vi "CorrectResponse.vi"(8 "error in (no error)":errorcluster, 11 "TrialBasedExperiment in":refnum<class "EyeCalibration.lvclass">) -> (0 "error out":errorcluster, 3 "TrialBasedExperiment out":refnum<class "EyeCalibration.lvclass">)   [LabVIEW 2014, in "EyeCalibration.lvclass"]
uses:
  EyeCalibration.lvclass
  Trial Based Experiment Statechart/MatlabExperiment/MatlabExperiment.lvclass
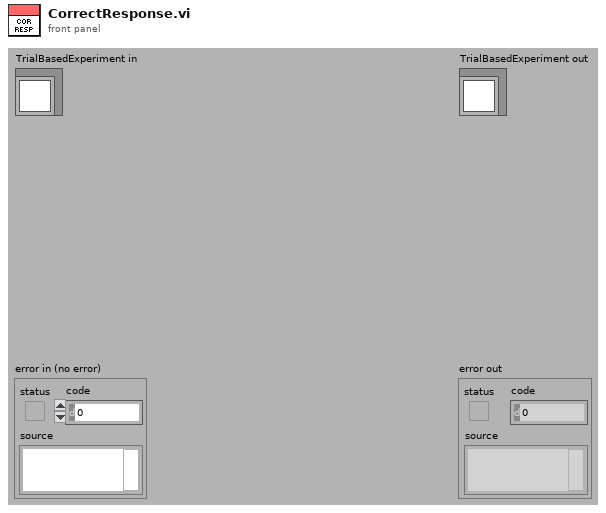
[diagram p1: front panel]
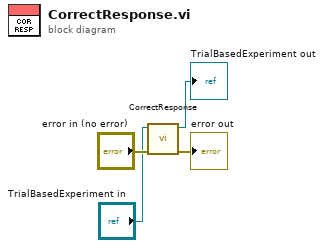
[diagram p0: block diagram]
diagram:
  n1 = call-parent "CorrectResponse.vi"("error in (no error)"="error in (no error)", "TrialBasedExperiment in"="TrialBasedExperiment in") -> ("error out"=→"error out":errorcluster, "TrialBasedExperiment out"=→"TrialBasedExperiment out":refnum<class "EyeCalibration.lvclass">)  [unwired: 8 in]
